vi "gRPC Client Test.vi"(8 "error in":errorcluster, 9 "relay names":string="K0", 10 "session name":string="<resource name>", 11 "resource name":string="<resource name>") -> (0 "error out":errorcluster, 3 "relay position":T1=10 items=["Open"=10, "Closed"=11])   [LabVIEW 2021, in "NI Switch Client.lvlib"]
uses:
  NI Switch Client.lvlib
  <instrlib>/niSwitch/niSwitch.llb/niSwitch Topologies.ctl
  <vilib>/Plug-In SDKs/Measurements/Measure Call Context/Measure Call Context.lvclass
  <instrlib>/niSwitch/niSwitch.llb/niSwitch Relay Position.ctl
  <instrlib>/niSwitch/niSwitch.llb/niSwitch Relay Action.ctl
  Session Factory/Client Wrapper Functions/niSwitch gRPC Device Server.ctl
  Session Factory/Session Factory.lvclass
  Session Management niSwitch.lvlib
  <vilib>/Plug-In SDKs/Clients/Session Management V1/Session Reservation/Session Reservation.lvclass
  <vilib>/Plug-In SDKs/Clients/Session Management V1/Session Reservation/Initialize and Close Session Behavior.ctl
  <vilib>/Plug-In SDKs/Measurements/Measure Call Context/Reserve Sessions - 1Pin.vi
  Initialize Sessions - 1Sess.vi
panel:
  out "relay position 2":T1=10 items=["Open"=10, "Closed"=11]
  in  "relay names 3":string
  in  "session name 2":string
  in  "relay names 2":string
  in  "error in 3":errorcluster
  out "measurement context out":refnum<class "Measure Call Context.lvclass">
  out "error out 3":errorcluster
  in  "measurement context in":refnum<class "Measure Call Context.lvclass">
  in  "pin or relay name":string
  in  "topology name":T2="Configured Topology"
  in  "error in 2":errorcluster
  out "error out 2":errorcluster
  # "Example in Disabled Structure"
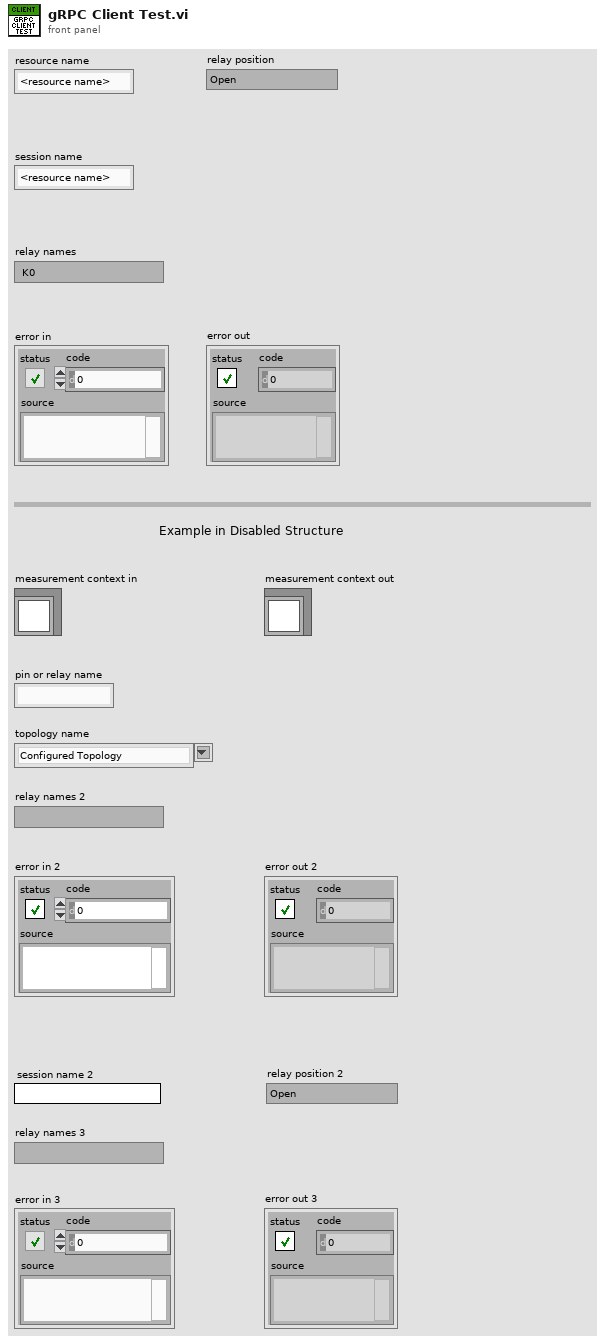
[diagram p1: front panel]
types:
  T1 = typedef "niSwitch Relay Position.ctl" = i32
  T2 = typedef "niSwitch Topologies.ctl" = string
  T3 = typedef "Session Management niSwitch.lvlib/Session Factory.lvclass/niSwitch gRPC Device Server.ctl" = cluster{"session name":string, "address (localhost)":string, "port (31763)":u32}
  T4 = typedef "niSwitch Relay Action.ctl" = i32
  T5 = typedef "NI Session Management V1 Client.lvlib/Session Reservation.lvclass/Initialize and Close Session Behavior.ctl" = enum16{"Auto", "Initialize and Close", "Attach and Detach", "Initialize and Detach", "Attach and Close"}
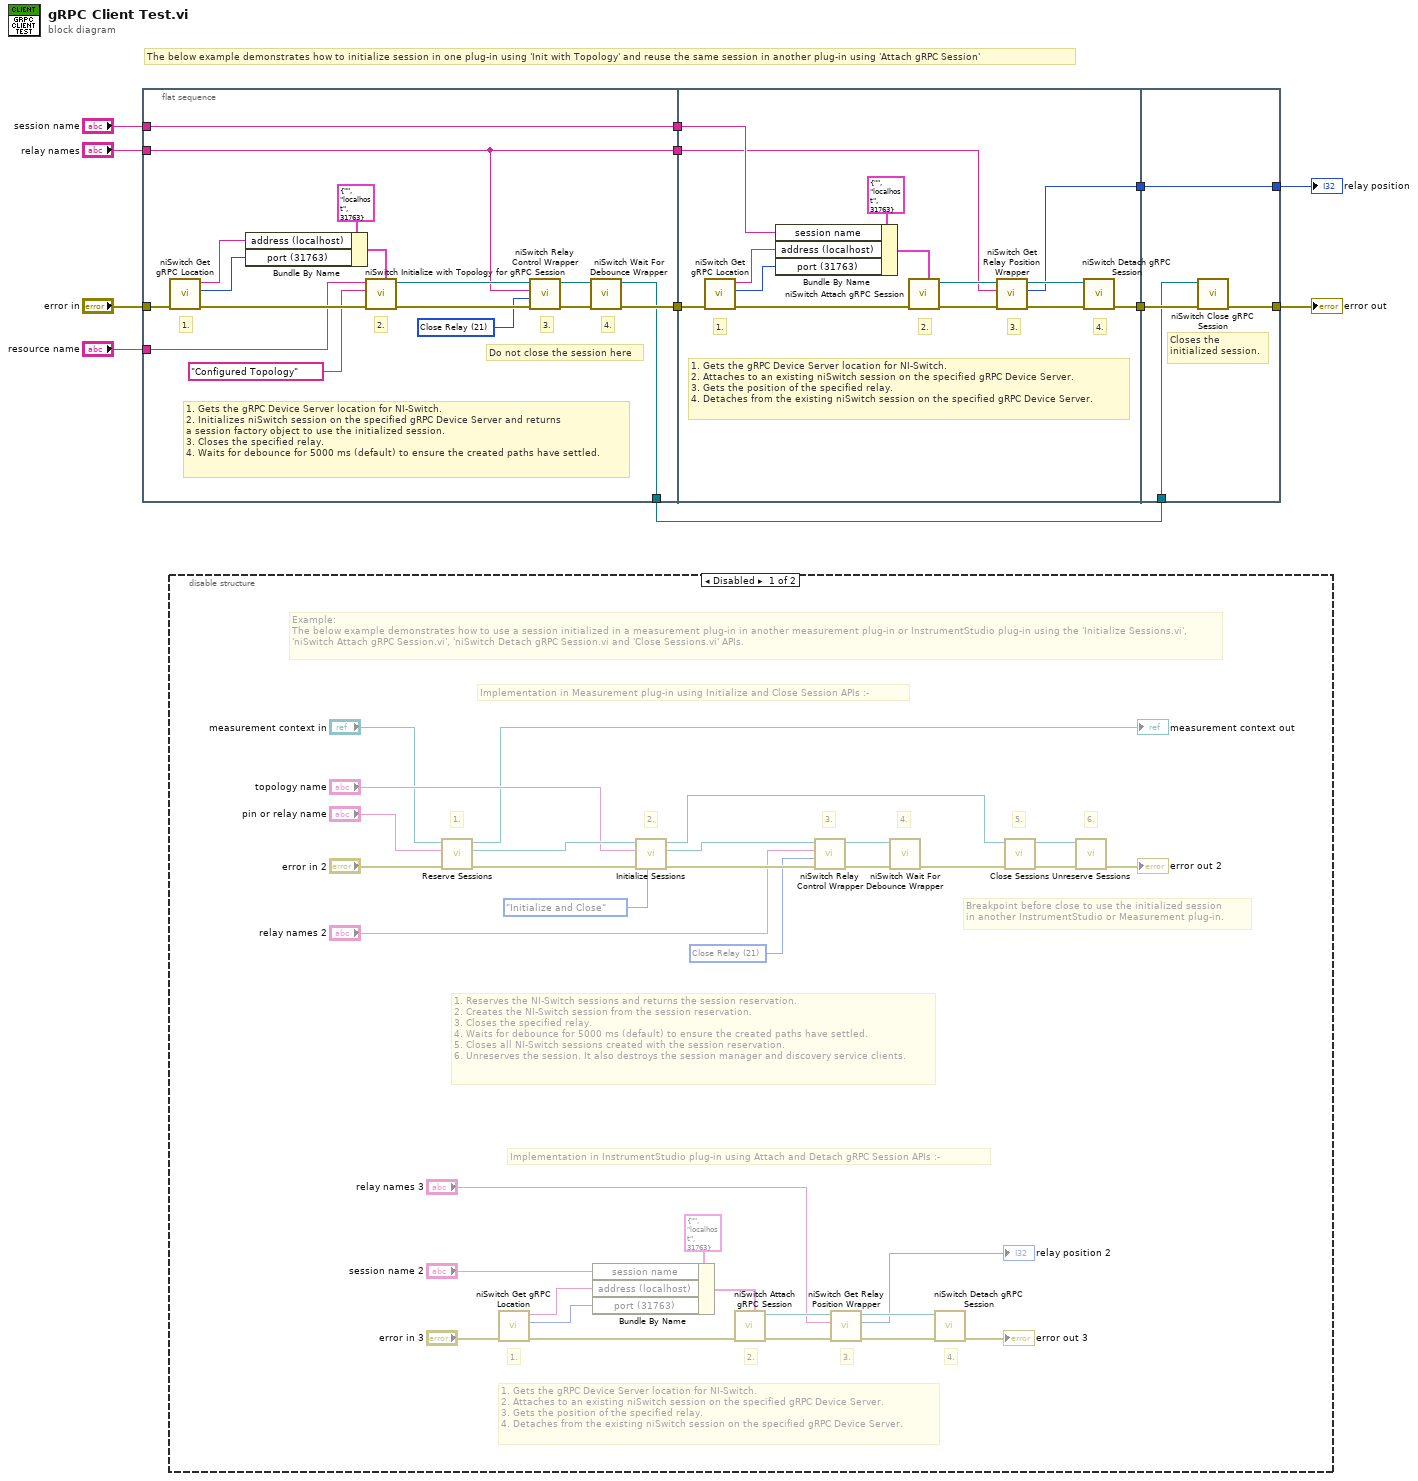
[diagram p0: block diagram]
diagram:
  # "The below example demonstrates how to initialize session in one plug-in using 'Init with Topology' and reuse the same session in another plug-in using 'Attach gRPC Session'"
  n1 = flat-sequence {
    tunnel: [w28] -> w12
    tunnel: [w15] -> w5
    tunnel: [w20] -> w10
    tunnel: "session name" -> [w20]
    tunnel: "relay names" -> [w17]
    tunnel: "error in" -> [w19]
    tunnel: [w17] -> w9
    tunnel: "resource name" -> [w14]
    tunnel: w12 -> [w41]
    tunnel: [w37] -> w11
    tunnel: w10 -> [w35]
    tunnel: w9 -> [w33]
    tunnel: [w31] -> w8
    tunnel: w11 -> [w47]
    tunnel: w5 -> [w44]
    tunnel: [w46] -> w7
    tunnel: w8 -> [w45]
    tunnel: [w45] -> w6
    frame #0 {
      w22 = T4 21 items=["Open Relay"=20, "Close Relay"=21] ("relay action (Close Relay)")
      # "Do not close the session here"
      # "4."
      # "3."
      # "2."
      # "1."
      # "1. Gets the gRPC Device Server location for NI-Switch.\n2. Initializes niSwitch session on the specified gRPC Device Server and returns\na session factory object to use the initialized session.\n3. Closes the specified relay.\n4. Waits for debounce for 5000 ms (default) to ensure the created paths have settled."
      n2 = call "niSwitch Get gRPC Location.vi"("error in"=w19) -> ("error out"=w21:errorcluster, "port"=w26:u32, "address"=w25:string)  [unwired: 8 in]
      n3 = Bundle By Name(cluster=T3 {"session name"="", "address (localhost)"="localhost", "port (31763)"=31763} ("gRPC options"), "address (localhost)"=w25, "port (31763)"=w26) -> (w16:T3)
      n4 = call "niSwitch Initialize with Topology for gRPC Session.vi"("gRPC options"=w16, "error in"=w21, "topology name"=T2 "Configured Topology", "resource name"=w14) -> ("error out"=w24:errorcluster, "session factory out"=w23:refnum<class "Session Factory.lvclass">)  [unwired: 6 in]
      n5 = call "niSwitch Relay Control Wrapper.vi"("error in"=w24, "relay action (Close Relay)"=w22, "relay names"=w17, "session factory in"=w23) -> ("error out"=w29:errorcluster, "session factory out"=w27:refnum<class "Session Factory.lvclass">)  [unwired: 6 in]
      n6 = call "niSwitch Wait For Debounce Wrapper.vi"("error in"=w29, "session factory in"=w27) -> ("error out"=w28:errorcluster, "session factory out"=w15:refnum<class "Session Factory.lvclass">)  [unwired: 8 in]
    }
    frame #1 {
      # "4."
      # "3."
      # "2."
      # "1."
      # "1. Gets the gRPC Device Server location for NI-Switch.\n2. Attaches to an existing niSwitch session on the specified gRPC Device Server.\n3. Gets the position of the specified relay.\n4. Detaches from the existing niSwitch session on the specified gRPC Device Server."
      n7 = call "niSwitch Get gRPC Location.vi"("error in"=w41) -> ("error out"=w40:errorcluster, "port"=w42:u32, "address"=w43:string)  [unwired: 8 in]
      n8 = Bundle By Name(cluster=T3 {"session name"="", "address (localhost)"="localhost", "port (31763)"=31763} ("gRPC options"), "session name"=w35, "address (localhost)"=w43, "port (31763)"=w42) -> (w30:T3)
      n9 = call "niSwitch Attach gRPC Session.vi"("gRPC options"=w30, "error in"=w40) -> ("error out"=w39:errorcluster, "session factory out"=w36:refnum<class "Session Factory.lvclass">)  [unwired: 8 in]
      n10 = call "niSwitch Get Relay Position Wrapper.vi"("error in"=w39, "relay name"=w33, "session factory in"=w36) -> ("error out"=w38:errorcluster, "position"=w31:T1, "session factory out"=w34:refnum<class "Session Factory.lvclass">)  [unwired: 6 in]
      n11 = call "niSwitch Detach gRPC Session.vi"("error in"=w38, "session factory in"=w34) -> ("error out"=w37:errorcluster)  [unwired: 9 in]
    }
    frame #2 {
      # "Closes the initialized session."
      n12 = call "niSwitch Close gRPC Session.vi"("error in"=w47, "session factory in"=w44) -> ("error out"=w46:errorcluster)  [unwired: 9 in]
    }
  }
  n13 = disable-structure shown="Disabled" {
    frame Disabled {
      w54 = T4 21 items=["Open Relay"=20, "Close Relay"=21] ("relay action (Close Relay)")
      # "6."
      # "5."
      # "4."
      # "3."
      # "2."
      # "1."
      # "4."
      # "3."
      # "2."
      # "1."
      # "1. Gets the gRPC Device Server location for NI-Switch.\n2. Attaches to an existing niSwitch session on the specified gRPC Device Server.\n3. Gets the position of the specified relay.\n4. Detaches from the existing niSwitch session on the specified gRPC Device Server."
      # "1. Reserves the NI-Switch sessions and returns the session reservation.\n2. Creates the NI-Switch session from the session reservation.\n3. Closes the specified relay.\n4. Waits for debounce for 5000 ms (default) to ensure the created paths have settled. \n5. Closes all NI-Switch sessions created with the session reservation.\n6. Unreserves the session. It also destroys the session manager and discovery service clients."
      # "Implementation in Measurement plug-in using Initialize and Close Session APIs :-"
      # "Breakpoint before close to use the initialized session\nin another InstrumentStudio or Measurement plug-in."
      # "Example:\nThe below example demonstrates how to use a session initialized in a measurement plug-in in another measurement plug-in or InstrumentStudio plug-in using the 'Initialize Sessions.vi', 'niSwitch Attach gRPC Session.vi', 'niSwitch Detach gRPC Session.vi and 'Close Sessions.vi' APIs."
      # "Implementation in InstrumentStudio plug-in using Attach and Detach gRPC Session APIs :-"
      n14 = call-poly <vilib>:"Reserve Sessions.vi"("error in"="error in 2", "pin or relay name"="pin or relay name", "measurement context in"="measurement context in") -> ("error out"=w79:errorcluster, "session reservation out"=w77:refnum<class "Session Reservation.lvclass">, "measurement context out"=→"measurement context out":refnum<class "Measure Call Context.lvclass">)  [unwired: 6 in]
      n15 = call "niSwitch Get gRPC Location.vi"("error in"="error in 3") -> ("error out"=w58:errorcluster, "port"=w67:u32, "address"=w66:string)  [unwired: 8 in]
      n16 = Bundle By Name(cluster=T3 {"session name"="", "address (localhost)"="localhost", "port (31763)"=31763} ("gRPC options"), "session name"="session name 2", "address (localhost)"=w66, "port (31763)"=w67) -> (w48:T3)
      n17 = call-poly "Initialize Sessions.vi"("initialize and close session behavior"=Initialize_and_Close_Session_Behavior."Initialize and Close", "error in"=w79, "topology name"="topology name", "session reservation in"=w77) -> ("error out"=w78:errorcluster, "session"=w57:refnum<class "Session Factory.lvclass">, "session reservation out"=w72:refnum<class "Session Reservation.lvclass">)  [unwired: 4 in, 1 out]
      n18 = call "niSwitch Attach gRPC Session.vi"("gRPC options"=w48, "error in"=w58) -> ("error out"=w59:errorcluster, "session factory out"=w65:refnum<class "Session Factory.lvclass">)  [unwired: 8 in]
      n19 = call "niSwitch Relay Control Wrapper.vi"("error in"=w78, "relay action (Close Relay)"=w54, "relay names"="relay names 2", "session factory in"=w57) -> ("error out"=w75:errorcluster, "session factory out"=w74:refnum<class "Session Factory.lvclass">)  [unwired: 6 in]
      n20 = call "niSwitch Get Relay Position Wrapper.vi"("error in"=w59, "relay name"="relay names 3", "session factory in"=w65) -> ("error out"=w60:errorcluster, "position"=→"relay position 2":T1, "session factory out"=w64:refnum<class "Session Factory.lvclass">)  [unwired: 6 in]
      n21 = call "niSwitch Wait For Debounce Wrapper.vi"("error in"=w75, "session factory in"=w74) -> ("error out"=w73:errorcluster)  [unwired: 8 in, 1 out]
      n22 = call "niSwitch Detach gRPC Session.vi"("error in"=w60, "session factory in"=w64) -> ("error out"=→"error out 3":errorcluster)  [unwired: 9 in]
      n23 = call <vilib>:"Close Sessions.vi"("error in"=w73, "session reservation in"=w72) -> ("error out"=w53:errorcluster, "session reservation out"=w71:refnum<class "Session Reservation.lvclass">)  [unwired: 8 in]
      n24 = call <vilib>:"Unreserve Sessions.vi"("error in"=w53, "session reservation in"=w71) -> ("error out"=→"error out 2":errorcluster)  [unwired: 9 in]
    }
    frame Enabled {
    }
  }
  "error out" <- w7
  "relay position" <- w6
